vi "run_auto VF_test .vi"(7 "Cluster":T2, 8 "error in (no error)":errorcluster) -> (0 "error out":errorcluster)   [LabVIEW 2019]
uses:
  core_dataRefCluster.ctl
  core_dataRef.ctl
  core_dataCluster.ctl
  instrument/instr_dataCluster.ctl
  gui/test_result_user_event.ctl
  core_autoMonitorDataCluster.ctl
  limits/report_mode.ctl
  <vilib>/Platform/TimedLoop/XDataNode/timing_clust.ctl
  <vilib>/Platform/TimedLoop/XDataNode/nitl_modes.ctl
  <vilib>/Platform/TimedLoop/XDataNode/wakeup.ctl
  <vilib>/Platform/TimedLoop/XDataNode/XDataNode.xnode
  <vilib>/Platform/TimedLoop/XDataNode/XDNodeRunTimeDep.lvlib
  instrument/Instrument.lvclass
panel:
  in  "user event out":T1
  in  "modbusData":refnum<notifier>
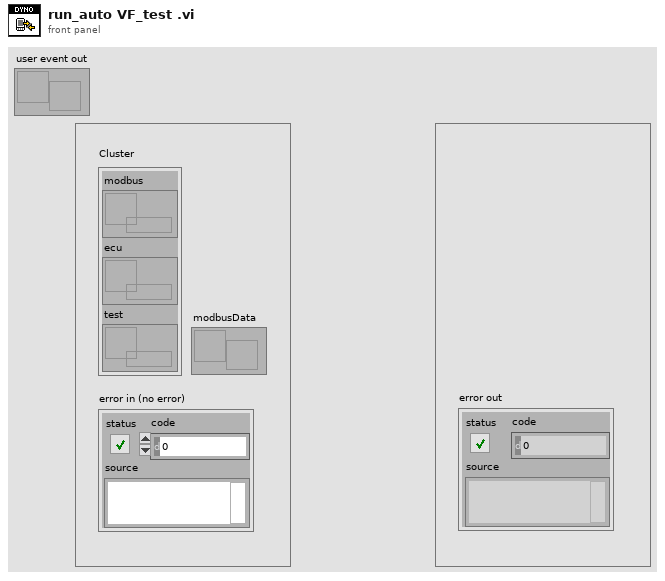
[diagram p1: front panel]
types:
  T1 = typedef "test_result_user_event.ctl" = refnum<user-event>
  T2 = typedef "core_dataRefCluster.ctl" = cluster{"modbus":T3, "ecu":T3, "test":T3}
  T3 = typedef "core_dataRef.ctl" = refnum<queue>
  T4 = typedef "report_mode.ctl" = enum16{"Initialize", "Save", "Close"}
  T5 = typedef "core_dataCluster.ctl" = cluster{"cmd":string, "data":variant}
  T6 = typedef "XDNodeRunTimeDep.lvlib/timing_clust.ctl" = cluster{"Expected End [f-1]":u64, "Actual End [f-1]":u64, "Finished Late? [f-1]":bool, "Expected End [i-1]":u64, "Actual End [i-1]":u64, "Finished Late? [i-1]":bool, "Expected Start [i]":u64, "Actual Start [i]":u64, "Expected Start [f]":u64, "Actual Start [f]":u64, "Source Name":string, "Structure Name":string, "Period":i64, "Deadline":i64, "Offset":i64, "Start":i64, "Priority":i32, "Timeout":i32, "Mode":T7, "Wakeup Reason":T8, "Error":errorcluster, "Source Type":string, "Secondary Source Type":string, "Global End Time":u64, "Global Start Time":u64, "Frame Duration":u64, "Iteration Duration":u64, "Assigned CPU":i32, "I/O Scan Engine Mode":u32}
  T7 = typedef "XDNodeRunTimeDep.lvlib/nitl_modes.ctl" = enum32{"No Change", "Process missed periods, maintain original phase", "Discard missed periods, maintain original phase", "Process missed periods, ignore original phase", "Discard missed periods, ignore original phase"}
  T8 = typedef "XDNodeRunTimeDep.lvlib/wakeup.ctl" = enum32{"Normal", "Aborted", "Asynchronous wakeup", "Timing source error", "Timed loop error", "Timeout"}
  T9 = typedef "limits_limitList.ctl" = cluster{"sec":i32, "spec":T10}
  T10 = typedef "limits_specs.ctl" = cluster{"torque":dbl, "lower_speed":dbl, "upper_speed":dbl, "input_power":dbl, "output_power":dbl, "efficiency":dbl}
  T11 = typedef "core_autoMonitorDataCluster.ctl" = cluster{"torque":dbl, "speed":dbl, "input power":dbl, "output power":dbl, "efficiency":dbl, "DC_power":dbl, "status":bool, "torque1":bool, "rpm1":bool, "Efficiency1":bool}
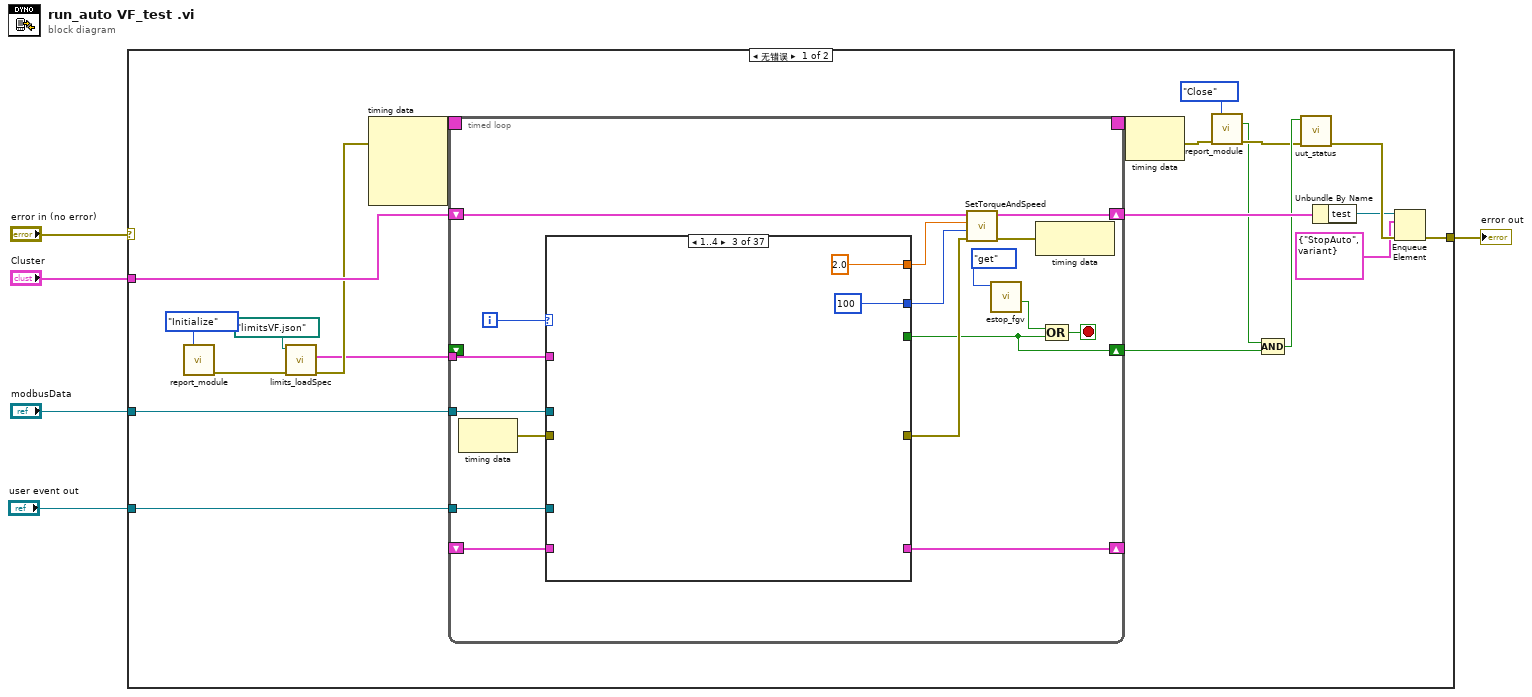
[diagram p0: block diagram]
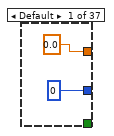
[diagram p2: hidden frame]
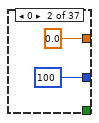
[diagram p3: hidden frame]
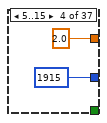
[diagram p4: hidden frame]
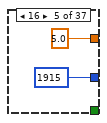
[diagram p5: hidden frame]
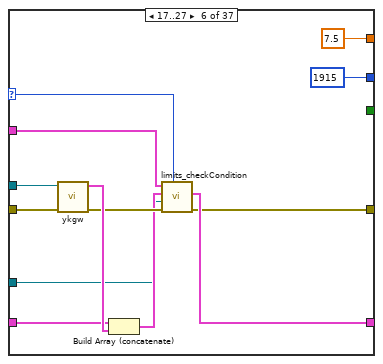
[diagram p6: hidden frame]
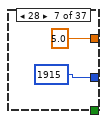
[diagram p7: hidden frame]
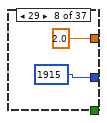
[diagram p8: hidden frame]
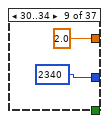
[diagram p9: hidden frame]
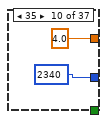
[diagram p10: hidden frame]
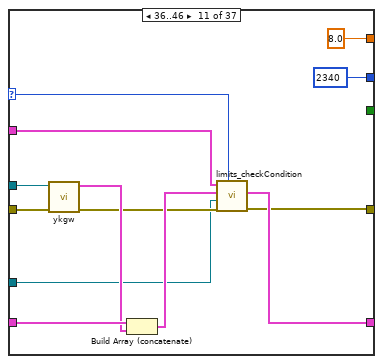
[diagram p11: hidden frame]
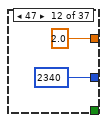
[diagram p12: hidden frame]
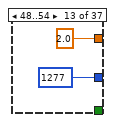
[diagram p13: hidden frame]
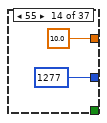
[diagram p14: hidden frame]
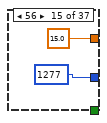
[diagram p15: hidden frame]
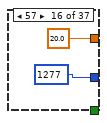
[diagram p16: hidden frame]
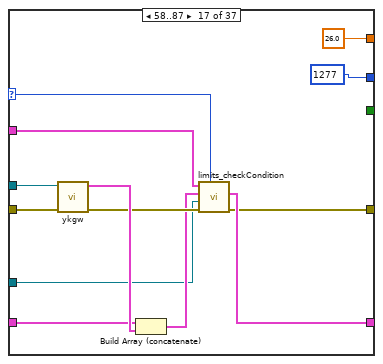
[diagram p17: hidden frame]
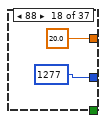
[diagram p18: hidden frame]
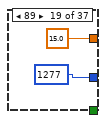
[diagram p19: hidden frame]
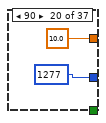
[diagram p20: hidden frame]
diagram:
  n1 = case shown="无错误" "error in (no error)" {
    selector: "error in (no error)" -> [_ w195]
    tunnel: "Cluster" -> [w19 _]
    tunnel: [w23 w195] -> w4
    tunnel: "modbusData" -> [w18 _]
    tunnel: "user event out" -> [w12 _]
    frame No Error {
      n2 = call "report_module.vi"("mode"=report_mode."Initialize") -> ("error out"=w10:errorcluster)  [unwired: 9 in, 5 out]
      n3 = call "limits_loadSpec.vi"("error in (no error)"=w10, "limits file"=path "limitsVF.json") -> ("error out"=w17:errorcluster, "test limits"=w16:T9[])  [unwired: 8 in]
      n4 = node-c288(w17) -> (w21:T6)  [unwired: 3 in]
      n5 = timed-loop {
        timing: w21 -> [_]
        timing-out: [_] -> w20
        shift-right: [w39] -> w25
        shift-left: w19 -> [w42]
        tunnel: w18 -> [w35]
        shift-right: [w32] -> _
        shift-left: _ -> [w31]
        tunnel: w16 -> [w30]
        tunnel: w12 -> [w27]
        shift-right: [w28] -> w13
        shift-left: _ -> [_]
        i -> [w43]
        stop <- w36 stop-if-true
        n6 = node-c288() -> (w34:errorcluster)  [unwired: 1 in]
        n7 = case shown="1..4" w43 {
          selector: w43 -> [_ _ _ _ _ w57 _ _ _ _ w83 _ _ _ _ _ w100 _ _ _ _ _ w123 _ w137 _ _ _ _ _ w166 _ _ _ _ _ _]
          tunnel: [sgl 0.0 ("Torque") sgl 0.0 ("Torque") sgl 2.0 ("Torque") sgl 2.0 ("Torque") sgl 5.0 ("Torque") sgl 7.5 ("Torque") sgl 5.0 ("Torque") sgl 2.0 ("Torque") sgl 2.0 ("Torque") sgl 4.0 ("Torque") sgl 8.0 ("Torque") sgl 2.0 ("Torque") sgl 2.0 ("Torque") sgl 10.0 ("Torque") sgl 15.0 ("Torque") sgl 20.0 ("Torque") sgl 26.0 ("Torque") sgl 20.0 ("Torque") sgl 15.0 ("Torque") sgl 10.0 ("Torque") sgl 2.0 ("Torque") sgl 2.0 ("Torque") sgl 3.7 ("Torque") sgl 9.5 ("Torque") sgl 9.5 ("Torque") sgl 3.7 ("Torque") sgl 2.0 ("Torque") sgl 2.0 ("Torque") sgl 10.0 ("Torque") sgl 15.0 ("Torque") sgl 20.0 ("Torque") sgl 15.0 ("Torque") sgl 10.0 ("Torque") sgl 2.0 ("Torque") sgl 2.0 ("Torque") sgl 0.0 ("Torque") sgl 0.0 ("Torque")] -> w37
          tunnel: [0 ("Speed") 100 ("Speed") 100 ("Speed") 1915 ("Speed") 1915 ("Speed") 1915 ("Speed") 1915 ("Speed") 1915 ("Speed") 2340 ("Speed") 2340 ("Speed") 2340 ("Speed") 2340 ("Speed") 1277 ("Speed") 1277 ("Speed") 1277 ("Speed") 1277 ("Speed") 1277 ("Speed") 1277 ("Speed") 1277 ("Speed") 1277 ("Speed") 1277 ("Speed") 3830 ("Speed") 3830 ("Speed") 3830 ("Speed") 3830 ("Speed") 3830 ("Speed") 3830 ("Speed") 2128 ("Speed") 2128 ("Speed") 2128 ("Speed") 2128 ("Speed") 2128 ("Speed") 2128 ("Speed") 2128 ("Speed") 100 ("Speed") 100 ("Speed") 0 ("Speed")] -> w40
          tunnel: [_ _ _ _ _ _ _ _ _ _ _ _ _ _ _ _ _ _ _ _ _ _ _ _ _ _ _ _ _ _ _ _ _ _ _ _ TRUE] -> w28
          tunnel: w35 -> [_ _ _ _ _ w64 _ _ _ _ w85 _ _ _ _ _ w107 _ _ _ _ _ w126 _ w139 _ _ _ _ _ w164 _ _ _ _ _ _]
          tunnel: w34 -> [_ _ _ _ _ w62 _ _ _ _ w84 _ _ _ _ _ w106 _ _ _ _ _ w122 _ w138 _ _ _ _ _ w163 _ _ _ _ _ _]
          tunnel: [_ _ _ _ _ w55 _ _ _ _ w76 _ _ _ _ _ w99 _ _ _ _ _ w124 _ w141 _ _ _ _ _ w160 _ _ _ _ _ _] -> w33
          tunnel: [_ _ _ _ _ w56 _ _ _ _ w78 _ _ _ _ _ w102 _ _ _ _ _ w125 _ w140 _ _ _ _ _ w161 _ _ _ _ _ _] -> w32
          tunnel: w31 -> [_ _ _ _ _ w61 _ _ _ _ w81 _ _ _ _ _ w104 _ _ _ _ _ w130 _ w145 _ _ _ _ _ w162 _ _ _ _ _ _]
          tunnel: w30 -> [_ _ _ _ _ w58 _ _ _ _ w82 _ _ _ _ _ w101 _ _ _ _ _ w127 _ w142 _ _ _ _ _ w165 _ _ _ _ _ _]
          tunnel: w27 -> [_ _ _ _ _ w54 _ _ _ _ w75 _ _ _ _ _ w98 _ _ _ _ _ w121 _ w136 _ _ _ _ _ w159 _ _ _ _ _ _]
          frame Default {
          }
          frame 0 {
          }
          frame 1..4 {
          }
          frame 5..15 {
          }
          frame 16 {
          }
          frame 17..27 {
            n8 = call "ykgw.vi"("error in (no error)"=w62, "modbusData"=w64) -> ("error out"=w60:errorcluster, "Cluster"=w63:T11)  [unwired: 8 in]
            n9 = Build Array (concatenate)(w61, w63) -> (w59:T11[])
            n10 = call "limits_checkCondition.vi"("Sec"=w57, "error in (no error)"=w60, "user event out"=w54, "Data in"=w59, "test limits"=w58) -> ("error out"=w55:errorcluster, "Data out"=w56:T11[])  [unwired: 5 in]
          }
          frame 28 {
          }
          frame 29 {
          }
          frame 30..34 {
          }
          frame 35 {
          }
          frame 36..46 {
            n11 = call "ykgw.vi"("error in (no error)"=w84, "modbusData"=w85) -> ("error out"=w77:errorcluster, "Cluster"=w80:T11)  [unwired: 8 in]
            n12 = Build Array (concatenate)(w81, w80) -> (w79:T11[])
            n13 = call "limits_checkCondition.vi"("Sec"=w83, "error in (no error)"=w77, "user event out"=w75, "Data in"=w79, "test limits"=w82) -> ("error out"=w76:errorcluster, "Data out"=w78:T11[])  [unwired: 5 in]
          }
          frame 47 {
          }
          frame 48..54 {
          }
          frame 55 {
          }
          frame 56 {
          }
          frame 57 {
          }
          frame 58..87 {
            n14 = call "ykgw.vi"("error in (no error)"=w106, "modbusData"=w107) -> ("error out"=w105:errorcluster, "Cluster"=w108:T11)  [unwired: 8 in]
            n15 = Build Array (concatenate)(w104, w108) -> (w103:T11[])
            n16 = call "limits_checkCondition.vi"("Sec"=w100, "error in (no error)"=w105, "user event out"=w98, "Data in"=w103, "test limits"=w101) -> ("error out"=w99:errorcluster, "Data out"=w102:T11[])  [unwired: 5 in]
          }
          frame 88 {
          }
          frame 89 {
          }
          frame 90 {
          }
          frame 91 {
          }
          frame 92..112 {
          }
          frame 113..123 {
            n17 = call "ykgw.vi"("error in (no error)"=w122, "modbusData"=w126) -> ("error out"=w131:errorcluster, "Cluster"=w129:T11)  [unwired: 8 in]
            n18 = Build Array (concatenate)(w130, w129) -> (w128:T11[])
            n19 = call "limits_checkCondition.vi"("Sec"=w123, "error in (no error)"=w131, "user event out"=w121, "Data in"=w128, "test limits"=w127) -> ("error out"=w124:errorcluster, "Data out"=w125:T11[])  [unwired: 5 in]
          }
          frame 124 {
          }
          frame 125..134 {
            n20 = call "ykgw.vi"("error in (no error)"=w138, "modbusData"=w139) -> ("error out"=w146:errorcluster, "Cluster"=w144:T11)  [unwired: 8 in]
            n21 = Build Array (concatenate)(w145, w144) -> (w143:T11[])
            n22 = call "limits_checkCondition.vi"("Sec"=w137, "error in (no error)"=w146, "user event out"=w136, "Data in"=w143, "test limits"=w142) -> ("error out"=w141:errorcluster, "Data out"=w140:T11[])  [unwired: 5 in]
          }
          frame 135 {
          }
          frame 136 {
          }
          frame 137..147 {
          }
          frame 148 {
          }
          frame 149 {
          }
          frame 150..165 {
            n23 = call "ykgw.vi"("error in (no error)"=w163, "modbusData"=w164) -> ("error out"=w168:errorcluster, "Cluster"=w169:T11)  [unwired: 8 in]
            n24 = Build Array (concatenate)(w162, w169) -> (w167:T11[])
            n25 = call "limits_checkCondition.vi"("Sec"=w166, "error in (no error)"=w168, "user event out"=w159, "Data in"=w167, "test limits"=w165) -> ("error out"=w160:errorcluster, "Data out"=w161:T11[])  [unwired: 5 in]
          }
          frame 166 {
          }
          frame 167 {
          }
          frame 168 {
          }
          frame 169..178 {
          }
          frame 179 {
          }
          frame 180 {
          }
        }
        n26 = call "SetTorqueAndSpeed.vi"("error in (no error)"=w33, "Speed"=w40, "Torque"=w37, "Cluster in"=w42) -> ("error out"=w41:errorcluster, "Cluster out"=w39:T2)  [unwired: 6 in]
        n27 = call "estop_fgv.vi"("Enum"=enum16{"set", "get"}."get") -> ("indicator"=w29:bool)  [unwired: 9 in, 1 out]
        n28 = node-c288(w41) -> ()  [unwired: 1 out]
        n29 = Compound Arithmetic op=OR ("复合运算")(w29, w28) -> (w36:bool)
      }
      n30 = node-c288(w20) -> (w8:errorcluster)
      n31 = call "report_module.vi"("mode"=report_mode."Close", "error in (no error)"=w8) -> ("Passed"=w6:bool, "error out"=w7:errorcluster)  [unwired: 8 in, 4 out]
      n32 = Compound Arithmetic op=AND(w6, w13) -> (w14:bool)
      n33 = call "uut_status.vi"("error in (no error)"=w7, "status"=w14) -> ("error out"=w26:errorcluster)  [unwired: 9 in]
      n34 = Unbundle By Name(w25) -> ("test"=w24:T3)
      n35 = Enqueue Element(queue=w24, element=T5 {"cmd"="StopAuto", "data"=variant}, error in (no error)=w26) -> (error out=w23:errorcluster)  [unwired: 1 in, 2 out]
    }
    frame Error {
    }
  }
  "error out" <- w4
